vi "svx_Colormap Set Axis Range.vi"(6 "State in":T1={"RefQueue"=refnum, "Properties/Undo"=refnum, "Bound"={"Width"=0, "Height"=0}, "Plot Area:Colors"={"FG Color"=11776947, "BG Color"=0}, "scale legend visible?"=FALSE, "graph palette visible?"=FALSE, "cursor palette visible?"=FALSE, "Ignore Array"=TRUE, "Smooth Update"=FALSE, "Z Scale"={"Z Scale.Scale Fit"=2, "Z Scale.Name Label.Text"="Amplitude", "Z Scale.Interpolate Color"=TRUE, "Visible"=TRUE, "Label Visible"=TRUE, "format string"="%#.2g", "Z Scale.Range"={"Minimum"=0.0, "Maximum"=500.0}}, "X Scale"={"X Scale.Scale Fit"=2, "X Scale.Offset and Multiplier"={"Offset"=0.0, "Multiplier"=1.0}, "X Scale.Name Label.Text"="Time", "X Scale.Range"={"Minimum"=0.0, "Maximum"=10.0}, "Visible"=TRUE, "Label Visible"=TRUE, "format string"="%#.2g"}, "Y Scale"={"Y Scale.Scale Fit"=2, "Y Scale.Offset and Multiplier"={"Offset"=0.0, "Multiplier"=1.0}, "Y Scale.Name Label.Text"="Frequency", "Y Scale.Range"={"Minimum"=0.0, "Maximum"=500.0}, "Visible"=TRUE, "Label Visible"=TRUE, "format string"="%#.2g"}, "Annotation List"=[], "Cursor List"=[], "Display Frequency Lines"=TRUE, "Display Order Lines"=TRUE, "Display Order text"=TRUE, "Display Frequency text"=TRUE, "Order Lineproperty"={"Line"={"Width"=1, "Style"=enum."Dash"}, "color"=0}, "Order Textproperty"={"Test size"=11, "color"=16777222, "background"=16777216}, "Orders"=[], "Frequency"=[], "Frequency Lineproperty"={"Line"={"Width"=1, "Style"=enum."Dash"}, "color"=0}, "Frequency Textproperty"={"Test size"=11, "color"=16777222, "background"=16777216}, "Display Order from Cursor"=FALSE, "Display Freq from Cursor"=FALSE, "Active Cursor"=0, "Selected Cursors"=[], "Cursor Move"=refnum, "Scale Range Change"=refnum}, 7 "axis selection":u16(ring) items=["X-Axis", "Y-Axis", "Z-Axis"], 10 "empty?":bool, 11 "Color Map in":refnum<vi>) -> (2 "Range changed?":bool, 3 "Color Map out":refnum<vi>, 4 "State out":T1={"RefQueue"=refnum, "Properties/Undo"=refnum, "Bound"={"Width"=0, "Height"=0}, "Plot Area:Colors"={"FG Color"=11776947, "BG Color"=0}, "scale legend visible?"=FALSE, "graph palette visible?"=FALSE, "cursor palette visible?"=FALSE, "Ignore Array"=TRUE, "Smooth Update"=FALSE, "Z Scale"={"Z Scale.Scale Fit"=2, "Z Scale.Name Label.Text"="Amplitude", "Z Scale.Interpolate Color"=TRUE, "Visible"=TRUE, "Label Visible"=TRUE, "format string"="%#.2g", "Z Scale.Range"={"Minimum"=0.0, "Maximum"=500.0}}, "X Scale"={"X Scale.Scale Fit"=2, "X Scale.Offset and Multiplier"={"Offset"=0.0, "Multiplier"=1.0}, "X Scale.Name Label.Text"="Time", "X Scale.Range"={"Minimum"=0.0, "Maximum"=10.0}, "Visible"=TRUE, "Label Visible"=TRUE, "format string"="%#.2g"}, "Y Scale"={"Y Scale.Scale Fit"=2, "Y Scale.Offset and Multiplier"={"Offset"=0.0, "Multiplier"=1.0}, "Y Scale.Name Label.Text"="Frequency", "Y Scale.Range"={"Minimum"=0.0, "Maximum"=500.0}, "Visible"=TRUE, "Label Visible"=TRUE, "format string"="%#.2g"}, "Annotation List"=[], "Cursor List"=[], "Display Frequency Lines"=TRUE, "Display Order Lines"=TRUE, "Display Order text"=TRUE, "Display Frequency text"=TRUE, "Order Lineproperty"={"Line"={"Width"=1, "Style"=enum."Dash"}, "color"=0}, "Order Textproperty"={"Test size"=11, "color"=16777222, "background"=16777216}, "Orders"=[], "Frequency"=[], "Frequency Lineproperty"={"Line"={"Width"=1, "Style"=enum."Dash"}, "color"=0}, "Frequency Textproperty"={"Test size"=11, "color"=16777222, "background"=16777216}, "Display Order from Cursor"=FALSE, "Display Freq from Cursor"=FALSE, "Active Cursor"=0, "Selected Cursors"=[], "Cursor Move"=refnum, "Scale Range Change"=refnum})   [LabVIEW 2017, in "SVX Colormap.xctl"]
uses:
  <vilib>/addons/_XControls/Colormap/SVX Colormap.xctl
  <vilib>/addons/_XControls/Colormap/subVIs/svx_Colormap State.ctl
  <vilib>/addons/_XControls/Colormap/TypeDef/svx_Colormap_InnerState.ctl
  <vilib>/addons/_XControls/Colormap/TypeDef/svx_Colormap_Event.ctl
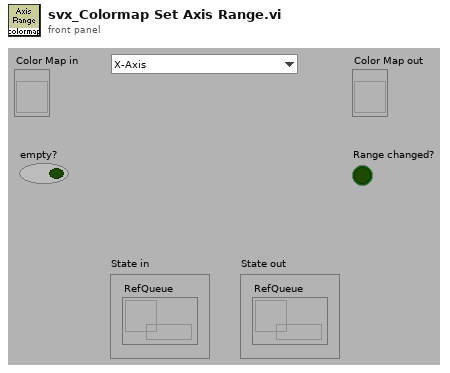
[diagram p1: front panel]
types:
  T1 = typedef "SVX Colormap.xctl/svx_Colormap State.ctl" = cluster{"RefQueue":refnum<queue>, "Properties/Undo":refnum<queue>, "Bound":cluster{"Width":u32, "Height":u32}, "Plot Area:Colors":cluster{"FG Color":u32, "BG Color":u32}, "scale legend visible?":bool, "graph palette visible?":bool, "cursor palette visible?":bool, "Ignore Array":bool, "Smooth Update":bool, "Z Scale":cluster{"Z Scale.Scale Fit":u8, "Z Scale.Name Label.Text":string, "Z Scale.Interpolate Color":bool, "Visible":bool, "Label Visible":bool, "format string":string, "Z Scale.Range":cluster{"Minimum":dbl, "Maximum":dbl}}, "X Scale":cluster{"X Scale.Scale Fit":u8, "X Scale.Offset and Multiplier":cluster{"Offset":dbl, "Multiplier":dbl}, "X Scale.Name Label.Text":string, "X Scale.Range":cluster{"Minimum":dbl, "Maximum":dbl}, "Visible":bool, "Label Visible":bool, "format string":string}, "Y Scale":cluster{"Y Scale.Scale Fit":u8, "Y Scale.Offset and Multiplier":cluster{"Offset":dbl, "Multiplier":dbl}, "Y Scale.Name Label.Text":string, "Y Scale.Range":cluster{"Minimum":dbl, "Maximum":dbl}, "Visible":bool, "Label Visible":bool, "format string":string}, "Annotation List":cluster{"Name":string, "Color":u32, "Style":u8, "Point Style":u8, "Name Visible":bool, "Allow Drag":bool, "Annotation Mode":u32, "Plot":i32, "Index":i32, "Position":cluster{"X":dbl, "Y":dbl}, "X Scale":u32, "Y Scale":u32, "Show Arrow":bool, "Lock Name":bool, "Plot Area":i32, "Label Offset":cluster{"X":dbl, "Y":dbl}}[], "Cursor List":cluster{"Name":string, "Color":u32, "Style":u8, "Point Style":u8, "Name Visible":bool, "Allow Drag":bool, "Cursor Mode":u32, "Plot":i32, "Index":i32, "Position":cluster{"X":dbl, "Y":dbl}, "X Scale":u32, "Y Scale":u32, "Watch Plots":i32[], "Watch All Plots":bool, "Plot Area":i32, "Label Offset":cluster{"X":dbl, "Y":dbl}}[], "Display Frequency Lines":bool, "Display Order Lines":bool, "Display Order text":bool, "Display Frequency text":bool, "Order Lineproperty":cluster{"Line":cluster{"Width":u16, "Style":enum32{"Solid", "Dash", "Dot", "DashDot", "DashDotDot"}}, "color":u32}, "Order Textproperty":cluster{"Test size":i16, "color":u32, "background":u32}, "Orders":dbl[], "Frequency":dbl[], "Frequency Lineproperty":cluster{"Line":cluster{"Width":u16, "Style":enum32{"Solid", "Dash", "Dot", "DashDot", "DashDotDot"}}, "color":u32}, "Frequency Textproperty":cluster{"Test size":i16, "color":u32, "background":u32}, "Display Order from Cursor":bool, "Display Freq from Cursor":bool, "Active Cursor":u32, "Selected Cursors":u32[], "Cursor Move":refnum<user-event>, "Scale Range Change":refnum<user-event>}
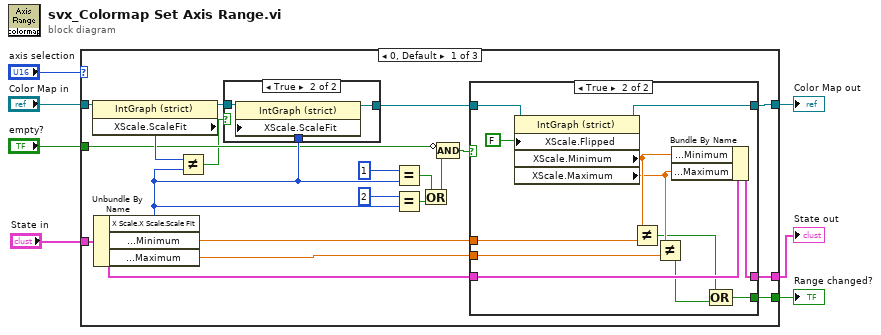
[diagram p0: block diagram]
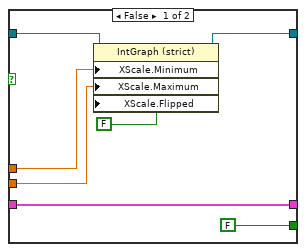
[diagram p3: hidden frame]
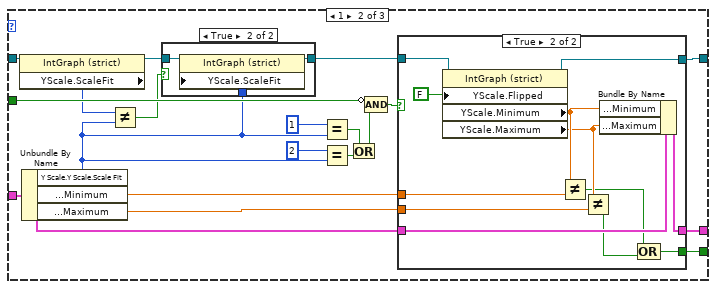
[diagram p4: hidden frame]
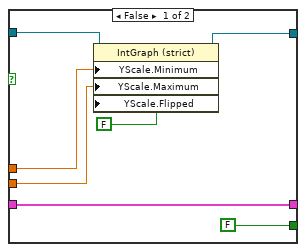
[diagram p6: hidden frame]
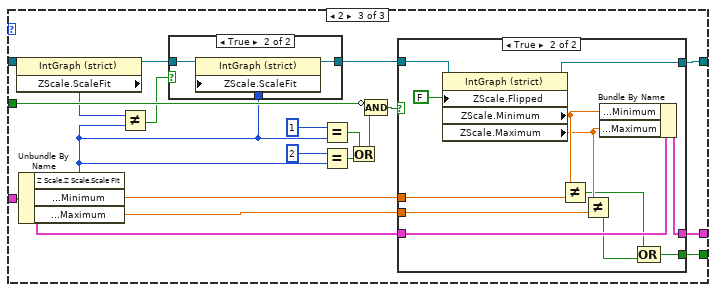
[diagram p7: hidden frame]
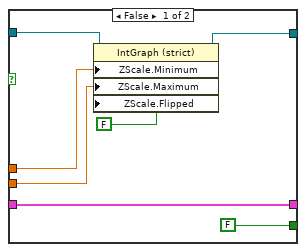
[diagram p9: hidden frame]
diagram:
  n1 = case shown="0, Default" "axis selection" {
    tunnel: "Color Map in" -> [w13 w53 w96]
    tunnel: "State in" -> [w26 w68 w110]
    tunnel: [w25 w67 w109] -> w1
    tunnel: "empty?" -> [w9 w62 w104]
    tunnel: [w15 w56 w98] -> w4
    tunnel: [w17 w58 w100] -> w3
    frame 0, Default {
      n2 = property class="IntGraph (strict)"(reference=w13) -> (reference out=w10:refnum<vi>, "XScale.ScaleFit"=w12:u8)  [unwired: 1 in, 1 out]
      n3 = Unbundle By Name(w26) -> ("X Scale.X Scale.Scale Fit"=w11:u8, "X Scale.X Scale.Range.Minimum"=w18:dbl, "X Scale.X Scale.Range.Maximum"=w16:dbl)
      n4 = Not Equal?(x=w12, y=w11) -> (x != y?=w8:bool)
      n5 = case shown="True" w8 {
        tunnel: [w27 w30] -> w14
        tunnel: w11 -> [_ w29]
        tunnel: w10 -> [w27 w28]
        frame False {
        }
        frame True {
          n6 = property class="IntGraph (strict)"(reference=w28, "XScale.ScaleFit"=w29) -> (reference out=w30:refnum<vi>)  [unwired: 1 in, 1 out]
        }
      }
      n7 = Equal?(x=u8 1, y=w11) -> (x = y?=w21:bool)
      n8 = Equal?(x=u8 2, y=w11) -> (x = y?=w22:bool)
      n9 = Or(x=w21, y=w22) -> (x .or. y?=w20:bool)
      n10 = Compound Arithmetic op=AND(invert w9, w20) -> (w19:bool)
      n11 = case shown="True" w19 {
        tunnel: w26 -> [w37 w48]
        tunnel: [w37 w47] -> w25
        tunnel: w18 -> [w34 w46]
        tunnel: [FALSE ("Range changed?") w40] -> w17
        tunnel: w14 -> [w35 w49]
        tunnel: w16 -> [w33 w44]
        tunnel: [w32 w39] -> w15
        frame False {
          n12 = property class="IntGraph (strict)"(reference=w35, "XScale.Minimum"=w34, "XScale.Maximum"=w33, "XScale.Flipped"=FALSE ("X Scale.Flipped")) -> (reference out=w32:refnum<vi>)  [unwired: 1 in, 1 out]
        }
        frame True {
          n13 = property class="IntGraph (strict)"(reference=w49, "XScale.Flipped"=FALSE ("X Scale.Flipped")) -> (reference out=w39:refnum<vi>, "XScale.Minimum"=w45:dbl, "XScale.Maximum"=w43:dbl)  [unwired: 1 in, 1 out]
          n14 = Not Equal?(x=w45, y=w46) -> (x != y?=w42:bool)
          n15 = Not Equal?(x=w43, y=w44) -> (x != y?=w41:bool)
          n16 = Bundle By Name(cluster=w48, "X Scale.X Scale.Range.Minimum"=w45, "X Scale.X Scale.Range.Maximum"=w43) -> (w47:T1)
          n17 = Compound Arithmetic op=OR(w42, w41) -> (w40:bool)
        }
      }
    }
    frame 1 {
      n18 = property class="IntGraph (strict)"(reference=w53) -> (reference out=w52:refnum<vi>, "YScale.ScaleFit"=w51:u8)  [unwired: 1 in, 1 out]
      n19 = Unbundle By Name(w68) -> ("Y Scale.Y Scale.Scale Fit"=w54:u8, "Y Scale.Y Scale.Range.Minimum"=w59:dbl, "Y Scale.Y Scale.Range.Maximum"=w57:dbl)
      n20 = Not Equal?(x=w51, y=w54) -> (x != y?=w50:bool)
      n21 = case shown="True" w50 {
        tunnel: [w69 w72] -> w55
        tunnel: w54 -> [_ w71]
        tunnel: w52 -> [w69 w70]
        frame False {
        }
        frame True {
          n22 = property class="IntGraph (strict)"(reference=w70, "YScale.ScaleFit"=w71) -> (reference out=w72:refnum<vi>)  [unwired: 1 in, 1 out]
        }
      }
      n23 = Equal?(x=u8 1, y=w54) -> (x = y?=w63:bool)
      n24 = Equal?(x=u8 2, y=w54) -> (x = y?=w64:bool)
      n25 = Or(x=w63, y=w64) -> (x .or. y?=w61:bool)
      n26 = Compound Arithmetic op=AND(invert w62, w61) -> (w60:bool)
      n27 = case shown="True" w60 {
        tunnel: w68 -> [w79 w90]
        tunnel: [w79 w89] -> w67
        tunnel: w59 -> [w76 w88]
        tunnel: [FALSE ("Range changed?") w82] -> w58
        tunnel: w55 -> [w77 w91]
        tunnel: w57 -> [w75 w86]
        tunnel: [w74 w81] -> w56
        frame False {
          n28 = property class="IntGraph (strict)"(reference=w77, "YScale.Minimum"=w76, "YScale.Maximum"=w75, "YScale.Flipped"=FALSE ("X Scale.Flipped")) -> (reference out=w74:refnum<vi>)  [unwired: 1 in, 1 out]
        }
        frame True {
          n29 = property class="IntGraph (strict)"(reference=w91, "YScale.Flipped"=FALSE ("X Scale.Flipped")) -> (reference out=w81:refnum<vi>, "YScale.Minimum"=w87:dbl, "YScale.Maximum"=w85:dbl)  [unwired: 1 in, 1 out]
          n30 = Not Equal?(x=w87, y=w88) -> (x != y?=w84:bool)
          n31 = Not Equal?(x=w85, y=w86) -> (x != y?=w83:bool)
          n32 = Bundle By Name(cluster=w90, "Y Scale.Y Scale.Range.Minimum"=w87, "Y Scale.Y Scale.Range.Maximum"=w85) -> (w89:T1)
          n33 = Compound Arithmetic op=OR(w84, w83) -> (w82:bool)
        }
      }
    }
    frame 2 {
      n34 = property class="IntGraph (strict)"(reference=w96) -> (reference out=w95:refnum<vi>, "ZScale.ScaleFit"=w93:u8)  [unwired: 1 in, 1 out]
      n35 = Unbundle By Name(w110) -> ("Z Scale.Z Scale.Scale Fit"=w94:u8, "Z Scale.Z Scale.Range.Minimum"=w101:dbl, "Z Scale.Z Scale.Range.Maximum"=w99:dbl)
      n36 = Not Equal?(x=w93, y=w94) -> (x != y?=w92:bool)
      n37 = case shown="True" w92 {
        tunnel: [w111 w114] -> w97
        tunnel: w95 -> [w111 w113]
        tunnel: w94 -> [_ w112]
        frame False {
        }
        frame True {
          n38 = property class="IntGraph (strict)"(reference=w113, "ZScale.ScaleFit"=w112) -> (reference out=w114:refnum<vi>)  [unwired: 1 in, 1 out]
        }
      }
      n39 = Equal?(x=u8 1, y=w94) -> (x = y?=w105:bool)
      n40 = Equal?(x=u8 2, y=w94) -> (x = y?=w106:bool)
      n41 = Or(x=w105, y=w106) -> (x .or. y?=w103:bool)
      n42 = Compound Arithmetic op=AND(invert w104, w103) -> (w102:bool)
      n43 = case shown="True" w102 {
        tunnel: w110 -> [w121 w132]
        tunnel: [w121 w131] -> w109
        tunnel: w101 -> [w118 w130]
        tunnel: [FALSE ("Range changed?") w124] -> w100
        tunnel: w97 -> [w119 w133]
        tunnel: w99 -> [w117 w128]
        tunnel: [w116 w123] -> w98
        frame False {
          n44 = property class="IntGraph (strict)"(reference=w119, "ZScale.Minimum"=w118, "ZScale.Maximum"=w117, "ZScale.Flipped"=FALSE ("X Scale.Flipped")) -> (reference out=w116:refnum<vi>)  [unwired: 1 in, 1 out]
        }
        frame True {
          n45 = property class="IntGraph (strict)"(reference=w133, "ZScale.Flipped"=FALSE ("X Scale.Flipped")) -> (reference out=w123:refnum<vi>, "ZScale.Minimum"=w129:dbl, "ZScale.Maximum"=w127:dbl)  [unwired: 1 in, 1 out]
          n46 = Not Equal?(x=w129, y=w130) -> (x != y?=w126:bool)
          n47 = Not Equal?(x=w127, y=w128) -> (x != y?=w125:bool)
          n48 = Bundle By Name(cluster=w132, "Z Scale.Z Scale.Range.Minimum"=w129, "Z Scale.Z Scale.Range.Maximum"=w127) -> (w131:T1)
          n49 = Compound Arithmetic op=OR(w126, w125) -> (w124:bool)
        }
      }
    }
  }
  "Color Map out" <- w4
  "Range changed?" <- w3
  "State out" <- w1
